vi "fpga_StepSize PI.vi"(0 "Crossing U[32.16]":fxp<+,32,16>, 5 "interpolation factor":u16=64, 9 "input valid":bool, 12 "ready for output":bool) -> (4 "Crossing[U64.16]":fxp<+,64,16> format="%.53g", 6 "Stepsize[U64.8]":fxp<+,64,8>, 10 "output valid":bool, 14 "ready for input":bool)   [LabVIEW 2011, in "NI_EP_Resample_FPGA.lvlib"]
uses:
  <vilib>/addons/Electrical Power/PQ/Resampling/NI_EP_Resample_FPGA.lvlib
  <vilib>/rvi/DataTransferAndStorage/Container/Common/niFpgaContainerState.ctl
  <vilib>/rvi/DataTransferAndStorage/Container/Common/niFpgaDataTypeControl.ctl
  <vilib>/rvi/DataTransferAndStorage/Container/Common/niFpgaContainerImplementationControl.ctl
  <vilib>/rvi/DataTransferAndStorage/Container/Common/niFpgaContainerArbitrationOptionsControl.ctl
  <vilib>/rvi/DataTransferAndStorage/Container/Common/niFpgaTransferTypeControl.ctl
  <vilib>/rvi/DataTransferAndStorage/Container/Common/niFpgaContainerInitializationParameters.ctl
  <vilib>/rvi/Memory/Memory_Types/niFpgaMemoryInterfaceConfiguration.ctl
  <vilib>/rvi/FIFO/Fifo_Types/niFpgaFifoControlLogicControl.ctl
  <vilib>/rvi/DataTransferAndStorage/Container/Common/niFpgaContainerMetaDataKey.ctl
  <vilib>/rvi/FXPMathLib/FxpSub/subVIs/nifxpmath_Sub_SimConfig.ctl
  <vilib>/fxp/LVFixedPointQuantizationPolicyTypeDef.ctl
  <vilib>/fxp/LVFixedPointOverflowPolicyTypeDef.ctl
  <vilib>/rvi/FXPMathLib/FxpDiv/subVIs/nifxpmath_Div_SimConfig.ctl
  <vilib>/rvi/FXPMathLib/FxpConvert/subVIs/nifxpmath_Convert_SimConfig.ctl
  <vilib>/rvi/DataTransferAndStorage/Container/Common/niFpgaContainerGetUniqueNameForEmu.vi
  <vilib>/rvi/DataTransferAndStorage/Container/Common/niFpgaContainerSetEmuInfo.vi
  <vilib>/rvi/eio/common/nirviEmuReportErrorAndStop.vi
  <vilib>/rvi/FIFO/Fifo_Resource/nirvififoEmulationSetSize.vi
  <vilib>/rvi/FXPMathLib/FxpSub/simVIs/DllFxpSubTemp_sub.vi
  <vilib>/rvi/FXPMathLib/FxpDiv/simVIs/DllFxpDivTemp_sub.vi
  <vilib>/rvi/FXPMathLib/FxpConvert/simVIs/DllFxpConvertTemp_sub.vi
  <vilib>/rvi/LocalResourceManager/LocalResourceManager.xnode
  <vilib>/rvi/DataTransferAndStorage/Container/XNode/niFpgaContainer.xnode
  <vilib>/rvi/FIFO/Fifo_Resource/nirvififoEmulationRead.vi
  <vilib>/rvi/FXPMathLib/basic elements/FxpDiscreteDelay/XNode/nifxpmath_DiscreteDelay.xnode
  <vilib>/rvi/FXPMathLib/FxpAdd/XNode/nifxpmath_Add.xnode
  <vilib>/rvi/FXPMathLib/FxpSub/XNode/nifxpmath_Sub.xnode
  <vilib>/rvi/FXPMathLib/FxpDiv/XNode/nifxpmath_Div.xnode
  <vilib>/rvi/FIFO/Fifo_Resource/nirvififoEmulationWrite.vi
  <vilib>/rvi/FXPMathLib/FxpConvert/XNode/nifxpmath_Convert.xnode
  <vilib>/rvi/FXPMathLib/sim/FxpSim.dll
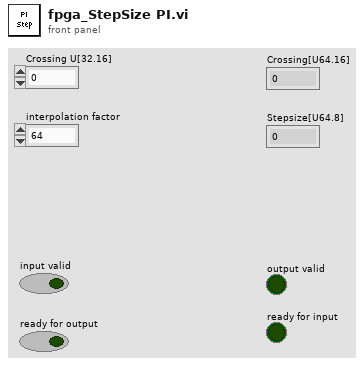
[diagram p1: front panel]
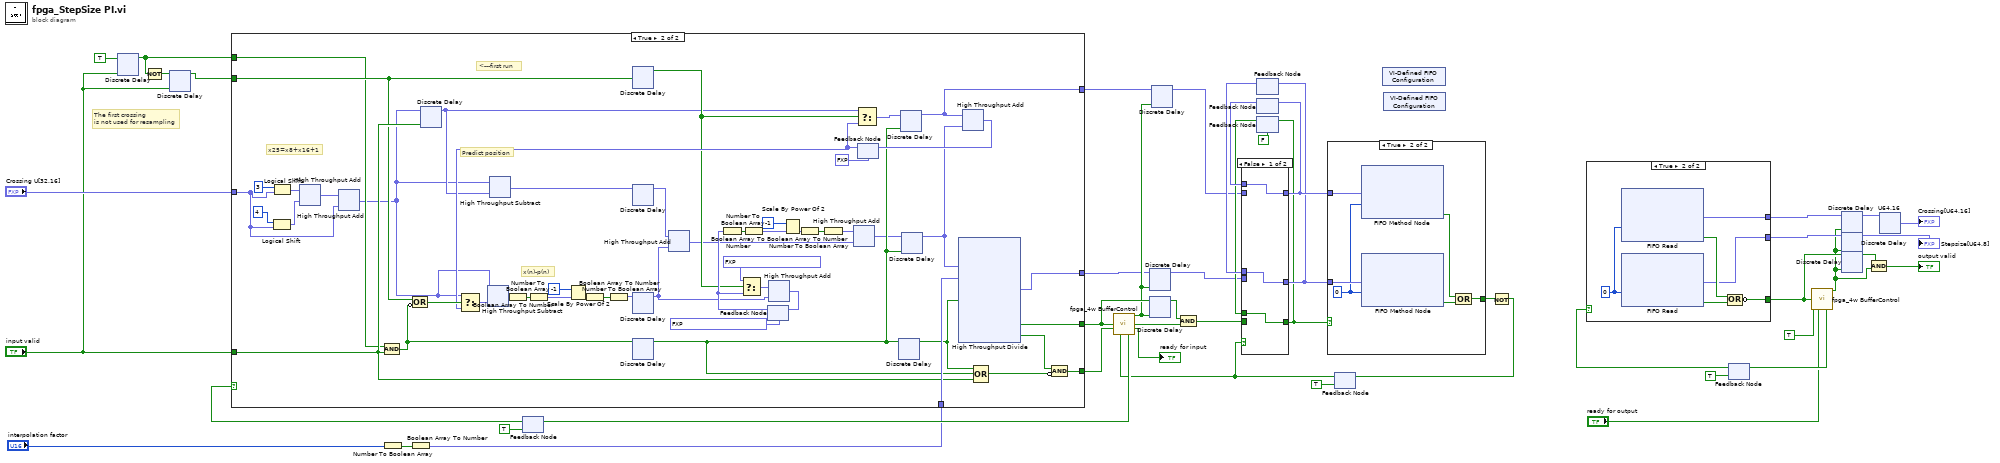
[diagram p0: block diagram]
diagram:
  # "The first crossing\nis not used for resampling"
  n1 = xnode "Discrete Delay"("D"=TRUE ("running"), "enable"="input valid") -> ("Q"=w3:bool)
  n2 = Not(x=w3) -> (.not. x?=w2:bool)
  n3 = xnode "Discrete Delay"("D"=w2, "enable"="input valid") -> ("Q"=w5:bool)
  n4 = Number To Boolean Array(number="interpolation factor") -> (Boolean array=w15:bool[])
  n5 = Boolean Array To Number(Boolean array=w15) -> (number=w11:fxp<+,16,16>)
  n6 = feedback #1(TRUE ("logic enable")) -> (w46:bool)
  n7 = case shown="True" w46 {
    tunnel: "input valid" -> [_ w75]
    tunnel: [_ w92] -> w18
    tunnel: [_ w86] -> w43
    tunnel: [_ w83] -> w44
    tunnel: "Crossing U[32.16]" -> [_ w50]
    tunnel: [_ w78] -> w22
    tunnel: w11 -> [_ w91]
    tunnel: w5 -> [_ w74]
    tunnel: w3 -> [_ w73]
    frame False {
    }
    frame True {
      # "x25=x8+x16+1"
      # "Predict position"
      # "x(n)-p(n)"
      # "<---first run"
      n8 = Logical Shift(y=i8 4, x=w50) -> (x << y=w52:fxp<+,32,16>)
      n9 = Logical Shift(y=i8 3, x=w50) -> (x << y=w53:fxp<+,32,16>)
      n10 = xnode "High Throughput Add"("x"=w53, "y"=w52) -> ("x+y"=w51:fxp<+,32,16>)
      n11 = xnode "High Throughput Add"("x"=w51, "y"=w50) -> ("x+y"=w49:fxp<+,32,16>)
      n12 = Compound Arithmetic op=AND(w73, w75) -> (w90:bool)
      n13 = Compound Arithmetic op=OR(w74, invert w90) -> (w79:bool)
      n14 = xnode "Discrete Delay"("D"=w49, "enable"=w75) -> ("Q"=w62:fxp<+,32,16>)
      n15 = xnode "High Throughput Subtract"("x"=w49, "y"=w62) -> ("x-y"=w61:fxp<+,32,16>)
      n16 = xnode "Discrete Delay"("D"=w74) -> ("Q"=w63:bool)
      n17 = xnode "Discrete Delay"("D"=w61) -> ("Q"=w60:fxp<+,32,16>)
      n18 = xnode "Discrete Delay"("D"=w90) -> ("Q"=w76:bool)
      n19 = feedback #2(fxp<+,32,16> 0.0 ("x+y")) -> (w88:fxp<+,32,16>)
      n20 = Number To Boolean Array(number=w88) -> (Boolean array=w99:bool[])
      n21 = Select(t=fxp<+,32,16> 0.0, s=w63, f=w88) -> (s? t:f=w89:fxp<+,32,16>)
      n22 = Boolean Array To Number(Boolean array=w99) -> (number=w96:fxp<+/-,32,16>)
      n23 = Scale By Power Of 2(n=-1, x=w96) -> (x*2^n=w94:fxp<+/-,32,16>)
      n24 = Number To Boolean Array(number=w94) -> (Boolean array=w95:bool[])
      n25 = Boolean Array To Number(Boolean array=w95) -> (number=w93:fxp<+,32,16>)
      n26 = feedback #3(fxp<+,32,16> 0.0 ("x+y")) -> (w77:fxp<+,32,16>)
      n27 = Select(t=w49, s=w79, f=w77) -> (s? t:f=w80:fxp<+,32,16>)
      n28 = xnode "High Throughput Subtract"("x"=w49, "y"=w80) -> ("x-y"=w64:fxp<+,32,16>)
      n29 = Number To Boolean Array(number=w64) -> (Boolean array=w67:bool[])
      n30 = Boolean Array To Number(Boolean array=w67) -> (number=w68:fxp<+/-,32,16>)
      n31 = Scale By Power Of 2(n=-1, x=w68) -> (x*2^n=w70:fxp<+/-,32,16>)
      n32 = Number To Boolean Array(number=w70) -> (Boolean array=w69:bool[])
      n33 = Boolean Array To Number(Boolean array=w69) -> (number=w65:fxp<+,32,16>)
      n34 = xnode "Discrete Delay"("D"=w65) -> ("Q"=w59:fxp<+,32,16>)
      n35 = xnode "High Throughput Add"("x"=w60, "y"=w59) -> ("x+y"=w58:fxp<+,32,16>)
      n36 = xnode "High Throughput Add"("x"=w89, "y"=w59) -> ("x+y"=w97:fxp<+,32,16>)
      n37 = feedback-in #2(w97) -> ()
      n38 = xnode "High Throughput Add"("x"=w93, "y"=w58) -> ("x+y"=w57:fxp<+,32,16>)
      n39 = Select(t=w62, s=w63, f=w77) -> (s? t:f=w82:fxp<+,32,16>)
      n40 = xnode "Discrete Delay"("D"=w76) -> ("Q"=w87:bool)
      n41 = xnode "Discrete Delay"("D"=w82, "enable"=w76) -> ("Q"=w78:fxp<+,32,16>)
      n42 = xnode "Discrete Delay"("D"=w57, "enable"=w76) -> ("Q"=w54:fxp<+,32,16>)
      n43 = xnode "High Throughput Divide"("x"=w54, "y"=w91, "input valid"=w87) -> ("x/y"=w92:fxp<+,64,8>, "output valid"=w86:bool, "ready for input"=w84:bool)  [unwired: 1 in]
      n44 = xnode "High Throughput Add"("x"=w78, "y"=w54) -> ("x+y"=w81:fxp<+,32,16>)
      n45 = feedback-in #3(w81) -> ()
      n46 = Compound Arithmetic op=OR(w87, w76, w75) -> (w85:bool)
      n47 = Compound Arithmetic op=AND(w84, invert w85) -> (w83:bool)
    }
  }
  n48 = feedback #4() -> (w40:fxp<+,64,8>)  [unwired: 1 in]
  n49 = feedback #5() -> (w41:fxp<+,32,16>)  [unwired: 1 in]
  n50 = feedback #6(FALSE) -> (w24:bool)
  n51 = feedback #7(TRUE) -> (w10:bool)
  n52 = call <vilib>:"fpga_4w BufferControl.vi"("DR"=w43, "RFI"=w44, "RFO"=w10) -> ("buff enable"=w23:bool, "output valid"=w27:bool, "ready for input"=→"ready for input":bool, "logic enable"=w47:bool)  [unwired: 9 in]
  n53 = feedback-in #1(w47) -> ()
  n54 = xnode "Discrete Delay"("D"=w18, "enable"=w23) -> ("Q"=w9:fxp<+,64,8>)
  n55 = xnode "Discrete Delay"("D"=w43, "enable"=w23) -> ("Q"=w42:bool)
  n56 = xnode "Discrete Delay"("D"=w22, "enable"=w23) -> ("Q"=w7:fxp<+,32,16>)
  n57 = Compound Arithmetic op=AND(w42, w27) -> (w8:bool)
  n58 = case shown="False" w10 {
    tunnel: w7 -> [_ w189]
    tunnel: w8 -> [_ w187]
    tunnel: w9 -> [_ w188]
    tunnel: [w186 w189] -> w39
    tunnel: w41 -> [w186 _]
    tunnel: [w185 w188] -> w38
    tunnel: w40 -> [w185 _]
    tunnel: [w184 w187] -> w26
    tunnel: w24 -> [w184 _]
    frame False {
    }
    frame True {
    }
  }
  n59 = feedback-in #4(w38) -> ()
  n60 = feedback-in #5(w39) -> ()
  n61 = feedback-in #6(w26) -> ()
  n62 = case shown="True" w26 {
    tunnel: w39 -> [_ w195]
    tunnel: w38 -> [_ w194]
    tunnel: [_ w190] -> w37
    frame False {
    }
    frame True {
      w193 = 0 ("Timeout")
      n63 = xnode ("FIFO Method Node")("Element"=w195, "Timeout"=w193) -> ("Timed Out?"=w191:bool)  [unwired: 1 in, 1 out]
      n64 = xnode ("FIFO Method Node")("Element"=w194, "Timeout"=w193) -> ("Timed Out?"=w192:bool)  [unwired: 1 in, 1 out]
      n65 = Compound Arithmetic op=OR(w191, w192) -> (w190:bool)
    }
  }
  n66 = xnode "VI-Defined FIFO Configuration"() -> ()  [unwired: 1 out]
  n67 = xnode "VI-Defined FIFO Configuration"() -> ()  [unwired: 1 out]
  n68 = Not(x=w37) -> (.not. x?=w1:bool)
  n69 = feedback-in #7(w1) -> ()
  n70 = feedback #8(TRUE ("logic enable")) -> (w34:bool)
  n71 = case shown="True" w34 {
    tunnel: [_ w199] -> w33
    tunnel: [_ w198] -> w30
    tunnel: [_ w196] -> w17
    frame False {
    }
    frame True {
      w197 = 0 ("Timeout")
      n72 = xnode ("FIFO Read")("Timeout"=w197) -> ("Element"=w196:fxp<+,32,16>, "Timed Out?"=w201:bool)  [unwired: 1 in, 1 out]
      n73 = xnode ("FIFO Read")("Timeout"=w197) -> ("Element"=w198:fxp<+,64,8>, "Timed Out?"=w200:bool)  [unwired: 1 in, 1 out]
      n74 = Compound Arithmetic op=OR(w201, w200) -> (invert w199:bool)
    }
  }
  n75 = call <vilib>:"fpga_4w BufferControl.vi"("DR"=w33, "RFI"=TRUE, "RFO"="ready for output") -> ("buff enable"=w19:bool, "logic enable"=w35:bool)  [unwired: 9 in, 2 out]
  n76 = feedback-in #8(w35) -> ()
  n77 = xnode "Discrete Delay"("D"=w17, "enable"=w19) -> ("Q"=w21:fxp<+,32,16>)
  n78 = xnode "Discrete Delay"("D"=w30, "enable"=w19) -> ("Q"=→"Stepsize[U64.8]":fxp<+,64,8>)
  n79 = xnode "Discrete Delay"("D"=w33, "enable"=w19) -> ("Q"=w32:bool)
  n80 = Compound Arithmetic op=AND(w32, w19) -> (→"output valid":bool)
  n81 = xnode "U64.16"("x"=w21) -> ("y"=→"Crossing[U64.16]":fxp<+,64,16>)
